vi "position setpoint(SubVI).vi"(0 "Position 2":dbl=300.0, 1 "Position":dbl=300.0, 5 "Instrument Ref":refnum<k24>, 6 "data":refnum<queue>, 7 "Delay":dbl, 9 "steps number":i32, 11 "Speed":i32=5 min=0 max=14, 12 "Resource In":refnum<visa-resource-name>, 13 "ch str":string, 15 "?":refnum<queue>) -> (8 "错误输出":errorcluster)   [LabVIEW 2019, in "old.lvlib"]
uses:
  old.lvlib
  SubVI.lvlib
  lib/QDInstrument.dll
  config.ctl
  <vilib>/NI/Modbus Library/API/Master/Modbus Master.lvclass
  Instrument.ctl
panel:
  out "数组":dbl[](array[numeric])
  # "(真是通道1，假是通道2)"
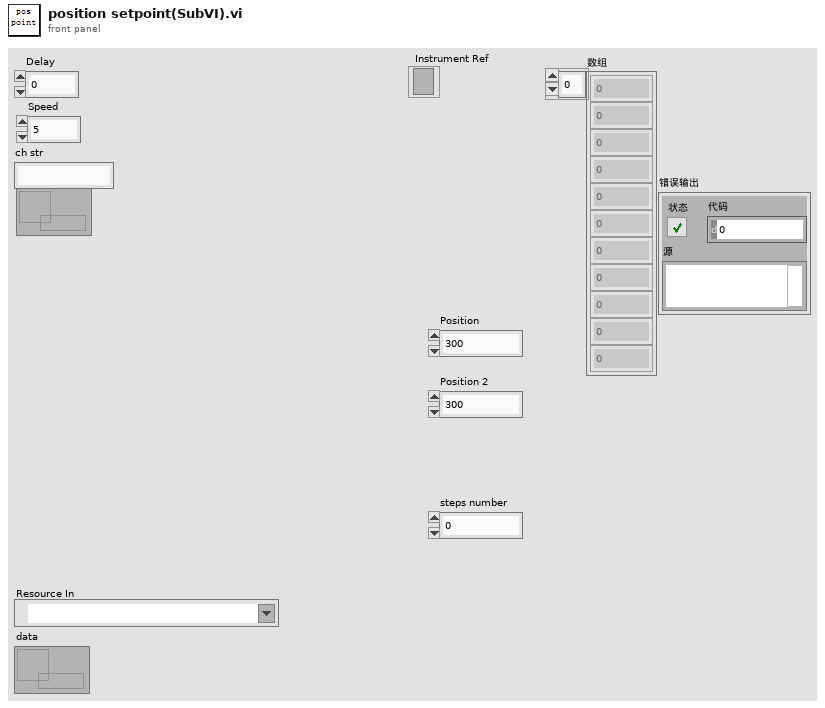
[diagram p1: front panel]
types:
  T1 = typedef "config.ctl" = cluster{"initialize":string, "6221":cluster{"6221 Resource":refnum<visa-resource-name>, "Delta status":bool}, "7001":cluster{"Ch":bool}, "SR830+6221":cluster{"source":u16, "阻抗":dbl, "量程入 4":i32, "量程入 3":i32, "量程入 2":i32, "量程入 1":i32, "电流":dbl, "SR830 2":bool, "SR830 3":bool, "SR830 4":bool, "SR830 1":bool, "VISA 1":refnum<visa-resource-name>, "VISA 2":refnum<visa-resource-name>, "VISA 3":refnum<visa-resource-name>, "VISA 4":refnum<visa-resource-name>, "量程":enum16{"量程每次测量会判定", "量程不变为设定值"}}, "2400":cluster{"2400":bool, "VISA":refnum<visa-resource-name>}, "ch":cluster{"ch str":string, "ch1":bool, "ch2":bool, "布尔":bool}, "error":bool, "数据文件路径":path, "log":cluster{"log路径":path, "log interval":dbl}, "Instrument":T2}
  T2 = typedef "Instrument.ctl" = cluster{"335 Resource":refnum<visa-resource-name>, "Input (0:A)":u16, "Instrument Type":i32, "quantum design":refnum<k24>, "Heater Output (1:1)":u16, "335state":refnum<vi>, "semaphore":T3, "TCP master instance":refnum<class "Modbus Master.lvclass">}
  T3 = typedef "Semaphore RefNum" = refnum<k1>
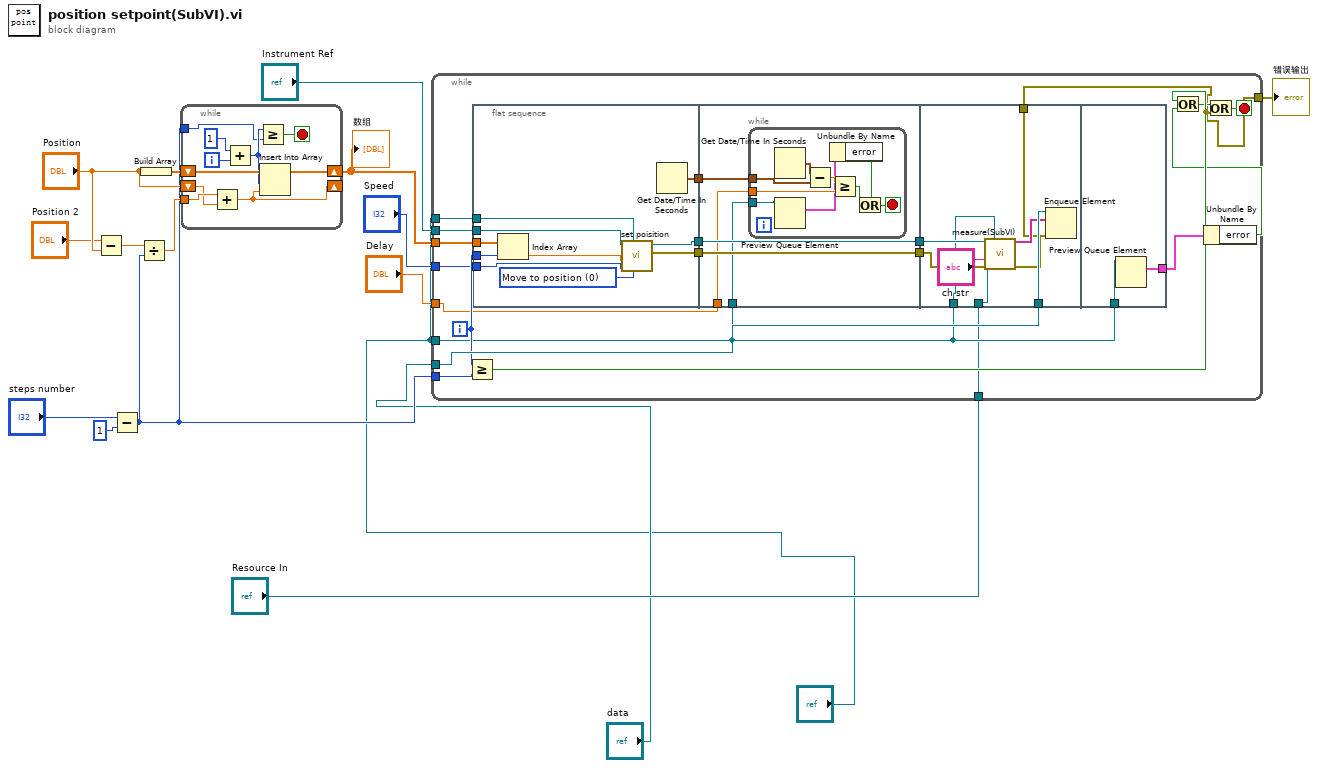
[diagram p0: block diagram]
diagram:
  n1 = Subtract(x="Position 2", y="Position") -> (x-y=w13:dbl)
  n2 = Subtract(x="steps number", y=1) -> (x-y=w6:i32)
  n3 = Divide(x=w13, y=w6) -> (x/y=w15:dbl)
  n4 = Build Array("Position") -> (w14:dbl[])
  n5 = while {
    shift-right: [w26] -> w11
    shift-left: w14 -> [w25]
    tunnel: w15 -> [w20]
    tunnel: w6 -> [w19]
    shift-right: [w18] -> _
    shift-left: "Position" -> [w17]
    i -> [w24]
    stop <- w21 stop-if-true
    n6 = Add(x=w20, y=w17) -> (x+y=w18:dbl)
    n7 = Add(x=1, y=w24) -> (x+y=w22:i32)
    n8 = Greater Or Equal?(x=w22, y=w19) -> (x >= y?=w21:bool)
    n9 = Insert Into Array(array=w25, index=w22, new element=w18) -> (w26:dbl[])
  }
  "数组" <- w11
  n10 = while {
    tunnel: w6 -> [w45]
    tunnel: "data" -> [w47]
    tunnel: "?" -> [w32]
    tunnel: "Instrument Ref" -> [w43]
    tunnel: w11 -> [w42]
    tunnel: "?" -> [w41]
    tunnel: [w29] -> w9
    tunnel: "Delay" -> [w33]
    tunnel: "Speed" -> [w31]
    tunnel: "Resource In" -> [w30]
    i -> [w44]
    stop <- w39 stop-if-true
    n11 = Greater Or Equal?(x=w44, y=w45) -> (x >= y?=w46:bool)
    n12 = flat-sequence {
      tunnel: [w48] -> w38
      tunnel: w44 -> [w55]
      tunnel: w43 -> [w54]
      tunnel: w42 -> [w56]
      tunnel: w41 -> [w49]
      tunnel: [w53] -> w36
      tunnel: [w52] -> w34
      tunnel: w31 -> [w51]
      tunnel: w38 -> [w62]
      tunnel: [w62] -> w37
      tunnel: w36 -> [w61]
      tunnel: [w61] -> w35
      tunnel: w34 -> [w60]
      tunnel: w33 -> [w59]
      tunnel: w32 -> [w58]
      tunnel: w37 -> [w80]
      tunnel: w47 -> [w79]
      tunnel: [w73] -> w29
      tunnel: w32 -> [w77]
      tunnel: w35 -> [w76]
      tunnel: w30 -> [w75]
      tunnel: w32 -> [w82]
      tunnel: [w81] -> w28
      frame #0 {
        w50 = u16 0 items=["Move to position", "Move to limit", "Redefine current position"] ("Mode")
        n13 = Index Array(array=w56, index=w55) -> (element=w57:dbl)
        n14 = call "set poisition.vi"("Mode"=w50, "config"=w49, "Slow down code\ndefault = 0"=w51, "Position (deg)"=w57, "Instrument Ref In"=w54) -> ("error out"=w53:errorcluster, "Instrument Ref Out"=w48:refnum<k24>)  [unwired: 3 in]
        n15 = Get Date/Time In Seconds() -> (seconds since 1Jan1904=w52:timestamp)
      }
      frame #1 {
        n16 = while {
          tunnel: w60 -> [w70]
          tunnel: w59 -> [w68]
          tunnel: w58 -> [w66]
          stop <- w65 stop-if-true
          n17 = Get Date/Time In Seconds() -> (seconds since 1Jan1904=w71:timestamp)
          n18 = Preview Queue Element(queue=w66) -> (element=w64:T1)  [unwired: 2 in, 3 out]
          n19 = Subtract(x=w71, y=w70) -> (x-y=w69:dbl)
          n20 = Unbundle By Name(w64) -> ("error"=w63:bool)
          n21 = Greater Or Equal?(x=w69, y=w68) -> (x >= y?=w67:bool)
          n22 = Or(x=w67, y=w63) -> (x .or. y?=w65:bool)
        }
      }
      frame #2 {
        n23 = call "measure(SubVI).vi"(0:w80, "config"=w77, 7:w75, "error in (no error)"=w76, 12:"ch str") -> ("data"=w78:string[], "error out"=w74:errorcluster)  [unwired: 9 in]
        n24 = Enqueue Element(queue=w79, element=w78, error in (no error)=w74) -> (error out=w73:errorcluster)  [unwired: 1 in, 2 out]
      }
      frame #3 {
        n25 = Preview Queue Element(queue=w82) -> (element=w81:T1)  [unwired: 2 in, 3 out]
      }
    }
    n26 = Unbundle By Name(w28) -> ("error"=w27:bool)
    n27 = Or(x=w46, y=w27) -> (x .or. y?=w40:bool)
    n28 = Or(x=w40, y=w29) -> (x .or. y?=w39:bool)
  }
  "错误输出" <- w9
